vi "modify.vi"(5 "operation":T1, 7 "section":T2, 8 "error in (no error)":errorcluster, 9 "index":i32, 10 "new text":string, 11 "id":string) -> (0 "error out":errorcluster)   [LabVIEW 2024, in "summary manager.lvlib"]
uses:
  summary manager.lvlib
  summary sections.ctl
  summary operations.ctl
  fgv actions.ctl
  <vilib>/Utility/error.llb/Error Cluster From Error Code.vi
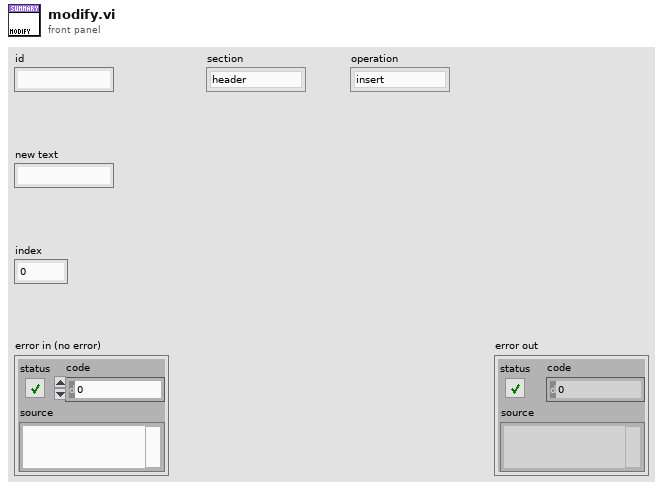
[diagram p1: front panel]
types:
  T1 = typedef "summary manager.lvlib/summary operations.ctl" = enum16{"insert", "replace", "delete"}
  T2 = typedef "summary manager.lvlib/summary sections.ctl" = enum16{"header", "body", "footer"}
  T3 = typedef "summary manager.lvlib/fgv actions.ctl" = enum16{"create", "get", "destroy"}
  T4 = typedef "summary manager.lvlib/collection type.ctl" = map{string, T5}
  T5 = typedef "summary manager.lvlib/entry type.ctl" = cluster{"summary control id":i32, "header":string[], "body":string[], "footer":string[]}
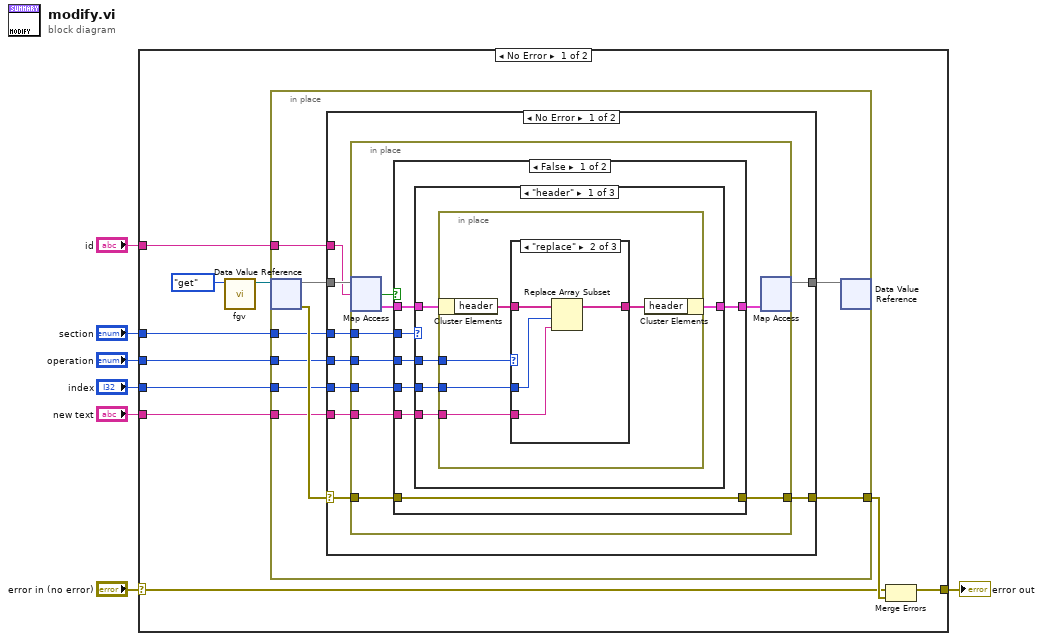
[diagram p0: block diagram]
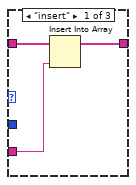
[diagram p2: hidden frame]
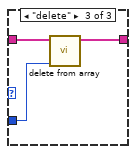
[diagram p3: hidden frame]
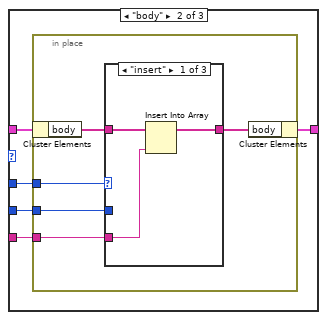
[diagram p4: hidden frame]
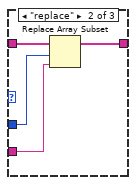
[diagram p5: hidden frame]
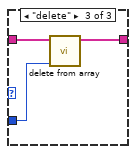
[diagram p6: hidden frame]
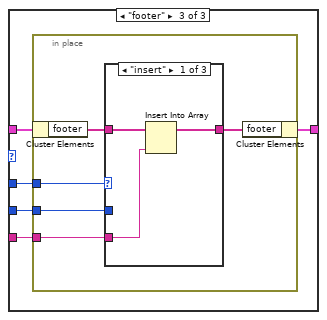
[diagram p7: hidden frame]
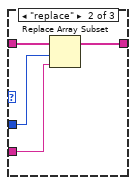
[diagram p8: hidden frame]
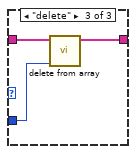
[diagram p9: hidden frame]
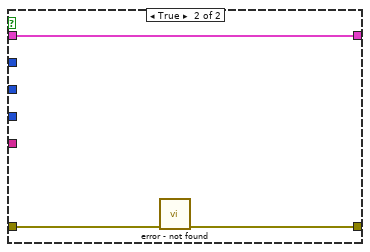
[diagram p10: hidden frame]
diagram:
  n1 = case shown="No Error" "error in (no error)" {
    selector: "error in (no error)" -> [w10 w117]
    tunnel: "new text" -> [w16 _]
    tunnel: "index" -> [w15 _]
    tunnel: "operation" -> [w14 _]
    tunnel: "section" -> [w13 _]
    tunnel: [w9 w117] -> w4
    tunnel: "id" -> [w8 _]
    frame No Error {
      n2 = call "fgv.vi"("action"=fgv_actions."get") -> ("dvr"=w12:refnum<data-value>)  [unwired: 9 in, 1 out]
      n3 = in-place {
        in-place-border: w13 -> [w23]
        in-place-border: w14 -> [w22]
        in-place-border: w15 -> [w21]
        in-place-border: w16 -> [w20]
        in-place-border: [w19] -> w17
        in-place-border: w8 -> [w18]
        n4 = in-place-dvr #1(w12) -> (w26:T4, w24:errorcluster)
        n5 = case shown="No Error" w24 {
          selector: w24 -> [w29 w116]
          tunnel: w26 -> [w35 w115]
          tunnel: [w34 w115] -> w25
          tunnel: w23 -> [w33 _]
          tunnel: w22 -> [w32 _]
          tunnel: w21 -> [w31 _]
          tunnel: w20 -> [w30 _]
          tunnel: [w28 w116] -> w19
          tunnel: w18 -> [w27 _]
          frame No Error {
            n6 = in-place {
              in-place-border: w33 -> [w42]
              in-place-border: w32 -> [w41]
              in-place-border: w31 -> [w40]
              in-place-border: w30 -> [w38]
              in-place-border: w29 -> [w37]
              in-place-border: [w36] -> w28
              n7 = in-place-map #2(w35, w27) -> (w43:T5, w44:bool)  [unwired: 1 in]
              n8 = case shown="False" w44 {
                tunnel: w43 -> [w49 w114]
                tunnel: w42 -> [w51 _]
                tunnel: w41 -> [w50 _]
                tunnel: w40 -> [w48 _]
                tunnel: [w47 w114] -> w39
                tunnel: w38 -> [w46 _]
                tunnel: w37 -> [w45 w113]
                tunnel: [w45 w112] -> w36
                frame False {
                  n9 = case shown="\"header\"" w51 {
                    tunnel: w50 -> [w56 w76 w96]
                    tunnel: w49 -> [w55 w75 w95]
                    tunnel: w48 -> [w54 w74 w94]
                    tunnel: [w53 w73 w93] -> w47
                    tunnel: w46 -> [w52 w72 w92]
                    frame "header" {
                      n10 = in-place {
                        in-place-border: w56 -> [w61]
                        in-place-border: w54 -> [w58]
                        in-place-border: w52 -> [w57]
                        n11 = in-place-cluster #3(w55) -> ("header"=w60:string[])
                        n12 = case shown="\"replace\"" w61 {
                          tunnel: w60 -> [w64 w68 w71]
                          tunnel: [w63 w67 w70] -> w59
                          tunnel: w58 -> [_ w66 w69]
                          tunnel: w57 -> [w62 w65 _]
                          frame "insert" {
                            n13 = Insert Into Array(array=w64, new element=w62) -> (w63:string[])  [unwired: 1 in]
                          }
                          frame "replace" {
                            n14 = Replace Array Subset(array=w68, new element=w65, index=w66) -> (w67:string[])
                          }
                          frame "delete" {
                            n15 = call "delete from array.vi"("index"=w69, "array in"=w71) -> ("array out"=w70:string[])  [unwired: 9 in]
                          }
                        }
                        n16 = in-place-cluster #3("header"=w59) -> (w53:T5)
                      }
                    }
                    frame "body" {
                      n17 = in-place {
                        in-place-border: w76 -> [w81]
                        in-place-border: w74 -> [w78]
                        in-place-border: w72 -> [w77]
                        n18 = in-place-cluster #4(w75) -> ("body"=w80:string[])
                        n19 = case shown="\"insert\"" w81 {
                          tunnel: w80 -> [w84 w88 w91]
                          tunnel: [w83 w87 w90] -> w79
                          tunnel: w78 -> [_ w86 w89]
                          tunnel: w77 -> [w82 w85 _]
                          frame "insert" {
                            n20 = Insert Into Array(array=w84, new element=w82) -> (w83:string[])  [unwired: 1 in]
                          }
                          frame "replace" {
                            n21 = Replace Array Subset(array=w88, new element=w85, index=w86) -> (w87:string[])
                          }
                          frame "delete" {
                            n22 = call "delete from array.vi"("index"=w89, "array in"=w91) -> ("array out"=w90:string[])  [unwired: 9 in]
                          }
                        }
                        n23 = in-place-cluster #4("body"=w79) -> (w73:T5)
                      }
                    }
                    frame "footer" {
                      n24 = in-place {
                        in-place-border: w96 -> [w101]
                        in-place-border: w94 -> [w98]
                        in-place-border: w92 -> [w97]
                        n25 = in-place-cluster #5(w95) -> ("footer"=w100:string[])
                        n26 = case shown="\"insert\"" w101 {
                          tunnel: w100 -> [w104 w108 w111]
                          tunnel: [w103 w107 w110] -> w99
                          tunnel: w98 -> [_ w106 w109]
                          tunnel: w97 -> [w102 w105 _]
                          frame "insert" {
                            n27 = Insert Into Array(array=w104, new element=w102) -> (w103:string[])  [unwired: 1 in]
                          }
                          frame "replace" {
                            n28 = Replace Array Subset(array=w108, new element=w105, index=w106) -> (w107:string[])
                          }
                          frame "delete" {
                            n29 = call "delete from array.vi"("index"=w109, "array in"=w111) -> ("array out"=w110:string[])  [unwired: 9 in]
                          }
                        }
                        n30 = in-place-cluster #5("footer"=w99) -> (w93:T5)
                      }
                    }
                  }
                }
                frame True {
                  n31 = call "error - not found.vi"("error in (no error)"=w113) -> ("error out"=w112:errorcluster)  [unwired: 10 in]
                }
              }
              n32 = in-place-map #2(w39) -> (w34:T4)  [unwired: 1 in, 2 out]
            }
          }
          frame Error {
          }
        }
        n33 = in-place-dvr #1(w25) -> ()  [unwired: 2 out]
      }
      n34 = Merge Errors(w10, w17) -> (w9:errorcluster)
    }
    frame Error {
    }
  }
  "error out" <- w4
